vi "TurnToAngle-C.vi"(11 "Params":string[][](array[string])) -> ()   [LabVIEW 2017]
uses:
  Framework/Robot Global Data.vi
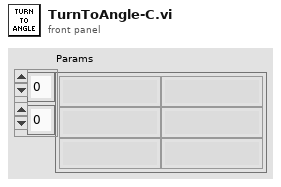
[diagram p1: front panel]
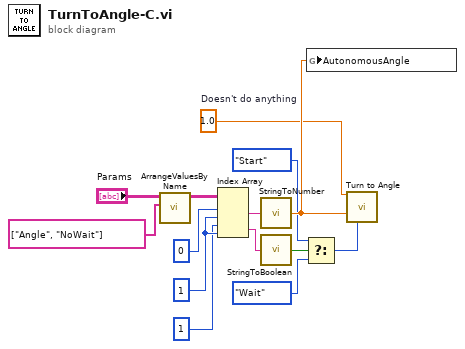
[diagram p0: block diagram]
diagram:
  w4 = 1
  w13 = 1.0  # Doesn't do anything
  n1 = call "ArrangeValuesByName.vi"("Names"=string[] ["Angle", "NoWait"], "Names/Values in"="Params") -> ("Names/Values Out"=w6:string[][])  [unwired: 9 in]
  n2 = Index Array(array=w6, index (row) #1=0, index (col) #1=w4, index (row) #2=1, index (col) #2=w4) -> (element #1=w2:string, element #2=w1:string)
  n3 = call "StringToNumber.vi"("String"=w2) -> ("Output"=w14:dbl)
  n4 = call "StringToBoolean.vi"("String"=w1) -> ("Output"=w12:bool)
  n5 = Select(t=enum16{"Start", "Wait"}."Start", s=w12, f=enum16{"Start", "Wait"}."Wait" ("Synchronication")) -> (s? t:f=w9:enum16{"Start", "Wait"})
  n6 = global write "Robot Global Data.vi" "AutonomousAngle"(w14) -> ()
  n7 = call "Turn to Angle.vi"("Speed"=w13, "Target Angle"=w14, "Synchronication"=w9) -> ()  [unwired: 12 in, 1 out]
